vi "Initialize.vi"(8 "error in (no error)":errorcluster, 9 "Reset (True)":bool=TRUE, 10 "ID Query (True)":bool=TRUE, 11 "VISA resource name":refnum<visa-resource-name>) -> (0 "error out":errorcluster, 3 "VISA resource name out":refnum<visa-resource-name>)   [LabVIEW 2012, in "Stanford Research 830.lvlib"]
doc: "Establishes communication with the instrument and optionally performs an instrument identification query and/or an instrument reset. It also places the instrument in a default state needed for other instrument driver operations. Therefore, call this VI before calling other instrument driver VIs for this instrument. Generally, you need to call the Initialize VI only once at the beginning of an application."
uses:
  Stanford Research 830.lvlib
panel:
  # "(c) 2006 National Instruments.  ALL RIGHTS RESERVED."
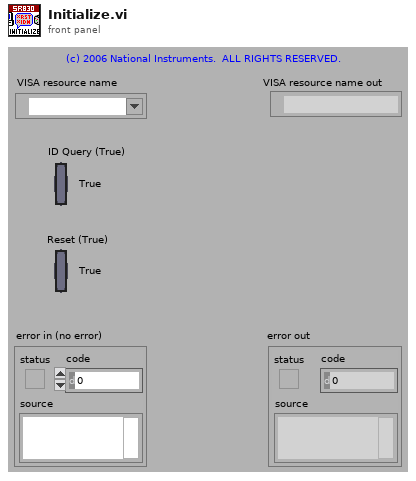
[diagram p1: front panel]
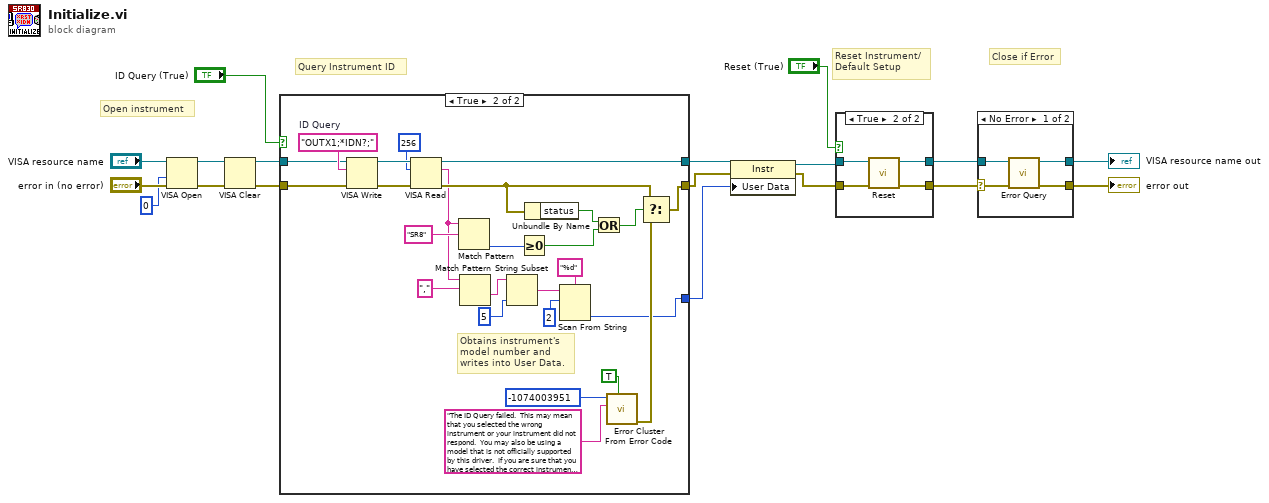
[diagram p0: block diagram]
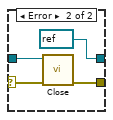
[diagram p2: hidden frame]
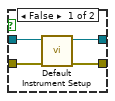
[diagram p3: hidden frame]
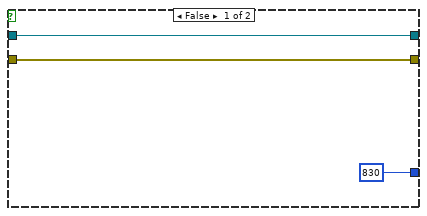
[diagram p4: hidden frame]
diagram:
  # "Close if Error"
  # "Query Instrument ID"
  # "Reset Instrument/\nDefault Setup"
  # "Open instrument"
  n1 = VISA Open(access mode=u32 0, error in (no error)="error in (no error)", VISA resource name="VISA resource name") -> (VISA resource name=w13:refnum<visa-resource-name>, error out=w12:errorcluster)  [unwired: 2 in]
  n2 = VISA Clear(VISA resource name=w13, error in (no error)=w12) -> (VISA resource name out=w7:refnum<visa-resource-name>, error out=w6:errorcluster)
  n3 = case shown="True" "ID Query (True)" {
    tunnel: [w20 w47] -> w3
    tunnel: [w21 w46] -> w4
    tunnel: w7 -> [w21 w31]
    tunnel: w6 -> [w20 w30]
    tunnel: [830 w22] -> w5
    frame False {
    }
    frame True {
      w41 = "OUTX1;*IDN?;"  # ID Query
      # "Obtains instrument's model number and writes into User Data."
      n4 = VISA Write(VISA resource name=w31, write buffer=w41, error in (no error)=w30) -> (VISA resource name out=w45:refnum<visa-resource-name>, error out=w44:errorcluster)  [unwired: 1 out]
      n5 = VISA Read(VISA resource name=w45, byte count=u32 256, error in (no error)=w44) -> (VISA resource name out=w46:refnum<visa-resource-name>, read buffer=w26:string, error out=w35:errorcluster)  [unwired: 1 out]
      n6 = Match Pattern(string=w26, regular expression="SR8") -> (offset past match=w36:i32)  [unwired: 1 in, 3 out]
      n7 = Match Pattern(string=w26, regular expression=",") -> (after substring=w27:string)  [unwired: 1 in, 3 out]
      n8 = String Subset(string=w27, length (rest)=5 ("length (rest)")) -> (substring=w25:string)  [unwired: 1 in]
      n9 = Greater Or Equal To 0?(x=w36) -> (x >= 0?=w33:bool)
      n10 = Unbundle By Name(w35) -> ("status"=w34:bool)
      n11 = Scan From String(format string="%d", input string=w25, initial scan location=2 ("offset")) -> (output 1=w22:i32)  [unwired: 2 in, 3 out]
      n12 = Or(x=w34, y=w33) -> (x .or. y?=w32:bool)
      n13 = call <vilib>:"Error Cluster From Error Code.vi"("show call chain? (False)"=TRUE, "error message (\"\")"="The ID Query failed.  This may mean that you selected the wrong instrument or your instrument did not respond.  You may also be using a model that is not officially supported by this driver.  If you are sure that you have selected the correct instrument and it is responding, try disabling the ID Query." ("Source (VI Name)"), "error code (0)"=-1074003951 ("Code")) -> ("error out"=w40:errorcluster)  [unwired: 6 in]
      n14 = Select(t=w35, s=w32, f=w40) -> (s? t:f=w47:errorcluster)
    }
  }
  n15 = property class="Instr"(reference=w4, error in=w3, "User Data"=w5) -> (reference out=w2:refnum<visa-resource-name>, error out=w1:errorcluster)
  n16 = case shown="True" "Reset (True)" {
    tunnel: w1 -> [w50 w52]
    tunnel: [w49 w55] -> w8
    tunnel: w2 -> [w51 w53]
    tunnel: [w48 w54] -> w9
    frame False {
      n17 = call "Default Instrument Setup.vi"("error in (no error)"=w50, "VISA resource name"=w51) -> ("error out"=w49:errorcluster, "VISA resource name out"=w48:refnum<visa-resource-name>)  [unwired: 8 in]
    }
    frame True {
      n18 = call "Reset.vi"("error in (no error)"=w52, "VISA resource name"=w53) -> ("error out"=w55:errorcluster, "VISA resource name out"=w54:refnum<visa-resource-name>)  [unwired: 8 in]
    }
  }
  n19 = case shown="No Error" w8 {
    selector: w8 -> [w56 w61]
    tunnel: w9 -> [w57 w62]
    tunnel: [w58 refnum<visa-resource-name> refnum ("VISA resource name out")] -> w11
    tunnel: [w59 w63] -> w10
    frame No Error {
      n20 = call "Error Query.vi"("error in (no error)"=w56, "VISA resource name"=w57) -> ("error out"=w59:errorcluster, "VISA resource name out"=w58:refnum<visa-resource-name>)  [unwired: 7 in, 1 out]
    }
    frame Error {
      n21 = call "Close.vi"("error in (no error)"=w61, "VISA resource name"=w62) -> ("error out"=w63:errorcluster)  [unwired: 9 in]
    }
  }
  "VISA resource name out" <- w11
  "error out" <- w10
